vi "Write Timestamp Configuration.vi"(8 "error in (no error)":errorcluster, 9 "Value":timestamp, 10 "Name":string, 11 "IniFileSection in":refnum<class "IniFileSection.lvclass">) -> (0 "error out":errorcluster, 3 "IniFileSection out":refnum<class "IniFileSection.lvclass">)   [LabVIEW 2017, in "IniFileSection.lvclass"]
uses:
  IniFileSection.lvclass
  IniFileSection.lvclass/IniFileSection.ctl
  <vilib>/Utility/config.llb/Write Key (String).vi
  <vilib>/Utility/config.llb/NI_LVConfig.lvlib
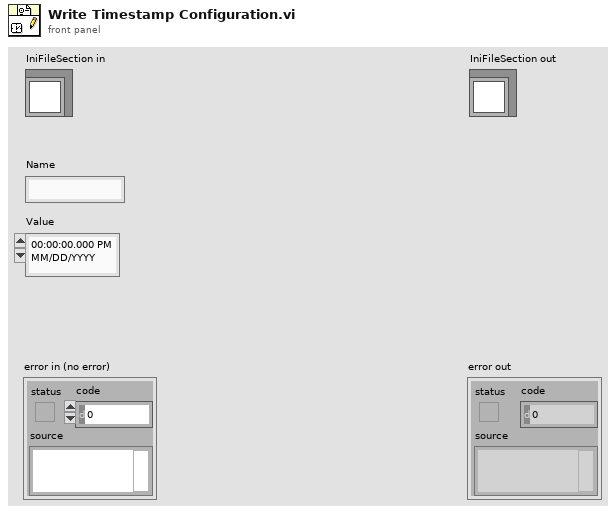
[diagram p1: front panel]
types:
  T1 = typedef "NI_LVConfig.lvlib/Config Data RefNum.ctl" = refnum<k1>
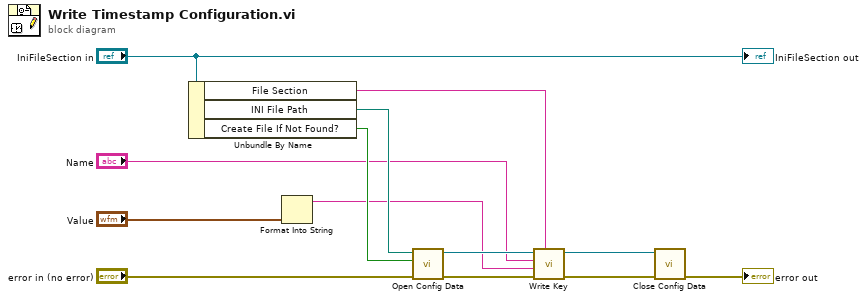
[diagram p0: block diagram]
diagram:
  n1 = Unbundle By Name("IniFileSection in") -> ("File Section"=w8:string, "INI File Path"=w9:path, "Create File If Not Found?"=w7:bool)
  n2 = Format Into String("Value") -> (resulting string=w1:string)  [unwired: 3 in, 1 out]
  n3 = call <vilib>:"Open Config Data.vi"("error in (no error)"="error in (no error)", "create file if necessary (T)"=w7, "configuration file path"=w9) -> ("error out"=w13:errorcluster, "refnum"=w11:T1)  [unwired: 6 in, 1 out]
  n4 = call-poly <vilib>:"Write Key.vi"("section"=w8, "error in (no error)"=w13, "value"=w1, "key"="Name", "refnum"=w11) -> ("error out"=w12:errorcluster, "refnum out"=w10:T1)  [unwired: 4 in, 1 out]
  n5 = call <vilib>:"Close Config Data.vi"("error in (no error)"=w12, "refnum"=w10) -> ("error out"=→"error out":errorcluster)  [unwired: 8 in, 1 out]
  "IniFileSection out" <- "IniFileSection in"
